vi "Read Timer Loop Timeout Period--constant.vi"() -> (0 "Read Timer Timeout":i32)   [LabVIEW 2024, in "EtherCAT Model.lvlib"]
uses:
  EtherCAT Model.lvlib
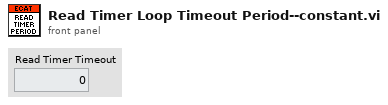
[diagram p1: front panel]
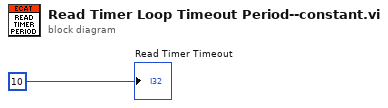
[diagram p0: block diagram]
diagram:
  "Read Timer Timeout" <- 10
